vi "Remove Attribute.vi"(8 "error in (no error)":errorcluster, 9 "Key":string, 10 "Object ID":i32=-1, 11 "Attributes in":refnum<class "Attributes.lvclass">) -> (0 "error out":errorcluster, 3 "Attributes out":refnum<class "Attributes.lvclass">)   [LabVIEW 2019, in "HierDAL Library.lvlib" / "Database.lvlib" / "Repositories.lvlib" / "Attributes.lvclass"]
uses:
  Attributes.lvclass
  Attributes.lvclass/Attributes.ctl
  Database Manager Class/Database Manager.lvclass
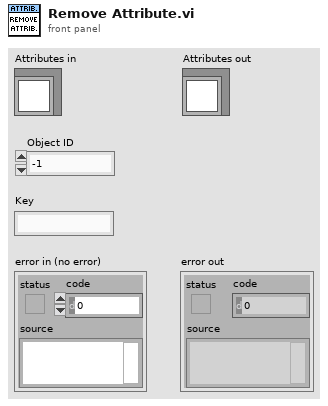
[diagram p1: front panel]
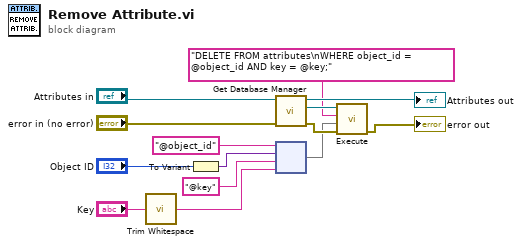
[diagram p0: block diagram]
diagram:
  n1 = call <vilib>:"Trim Whitespace.vi"("string"="Key") -> ("trimmed string"=w9:string)  [unwired: 1 in]
  n2 = To Variant(anything="Object ID") -> (Variant=w4:variant)
  n3 = call "Get Database Manager.vi"("error in (no error)"="error in (no error)", "Attributes in"="Attributes in") -> ("error out"=w12:errorcluster, "Database Manager"=w11:refnum<class "Database Manager.lvclass">, "Attributes out"=→"Attributes out":refnum<class "Attributes.lvclass">)  [unwired: 7 in]
  n4 = node("@object_id" ("key"), w4, "@key" ("key"), w9) -> (w5:map{string, variant})
  n5 = call-dynamic "Execute.vi"("error in (no error)"=w12, "Parameters"=w5, "Query"="DELETE FROM attributes\nWHERE object_id = @object_id AND key = @key;", "Database Manager in"=w11) -> ("error out"=→"error out":errorcluster)  [unwired: 5 in, 2 out]
